vi "CRYPick string arrays to save.vi"(8 "Axes":cluster{"x":bool, "y":bool, "z":bool}, 9 "Layout":enum16{"rows", "columns"}(ring), 10 "Delimiter":string, 11 "Spreadsheet string":string) -> (3 "Spreadsheet string out":string)   [LabVIEW 2013]
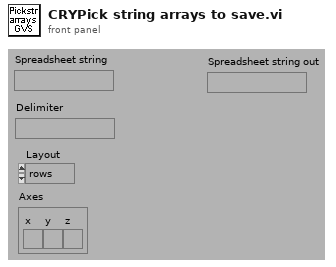
[diagram p1: front panel]
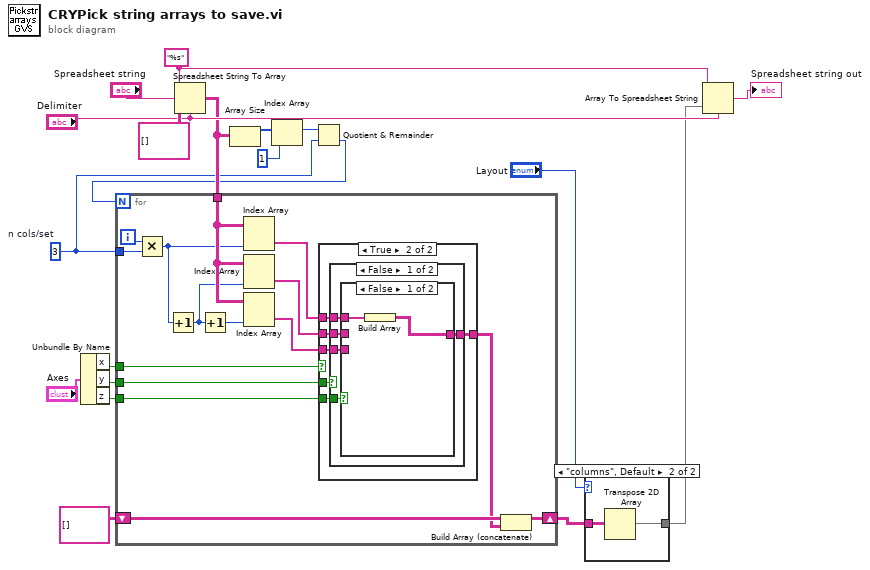
[diagram p0: block diagram]
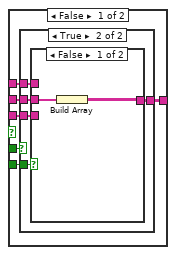
[diagram p3: hidden frame]
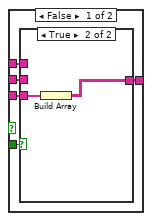
[diagram p4: hidden frame]
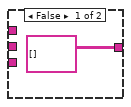
[diagram p5: hidden frame]
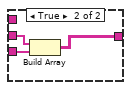
[diagram p6: hidden frame]
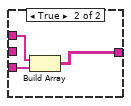
[diagram p7: hidden frame]
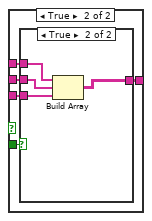
[diagram p8: hidden frame]
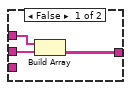
[diagram p9: hidden frame]
diagram:
  w5 = 3  # n cols/set
  w18 = "%s"
  n1 = Unbundle By Name("Axes") -> ("x"=w13:bool, "y"=w12:bool, "z"=w11:bool)
  n2 = Spreadsheet String To Array(delimiter (Tab)="Delimiter", format string=w18, spreadsheet string="Spreadsheet string", array type (2D Dbl)=string[][] []) -> (array=w7:string[][])
  n3 = Array Size(array=w7) -> (size(s)=w9:i32[])
  n4 = Index Array(array=w9, index=1 ("Index")) -> (element=w8:i32)
  n5 = Quotient & Remainder(x=w8, y=w5) -> (floor(x/y)=w6:i32)  [unwired: 1 out]
  n6 = for {
    N: w6 -> [_]
    tunnel: w7 -> [w34]
    tunnel: w13 -> [w30]
    tunnel: w12 -> [w29]
    tunnel: w11 -> [w28]
    tunnel: w5 -> [w25]
    shift-right: [w22] -> w3
    shift-left: string[][] [] -> [w21]
    i -> [w24]
    n7 = Multiply(x=w24, y=w25) -> (x*y=w23:i32)
    n8 = Increment(x=w23) -> (x+1=w26:i32)
    n9 = Increment(x=w26) -> (x+1=w27:i32)
    n10 = Index Array(array=w34, index (col)=w23) -> (element=w33:string[])  [unwired: 1 in]
    n11 = Index Array(array=w34, index (col)=w26) -> (element=w32:string[])  [unwired: 1 in]
    n12 = Index Array(array=w34, index (col)=w27) -> (element=w31:string[])  [unwired: 1 in]
    n13 = case shown="True" w30 {
      tunnel: w29 -> [w40 w64]
      tunnel: w28 -> [w39 w63]
      tunnel: w33 -> [w38 w62]
      tunnel: w32 -> [w37 w61]
      tunnel: w31 -> [w36 w60]
      tunnel: [w35 w59] -> w20
      frame False {
        n14 = case shown="True" w40 {
          tunnel: w39 -> [w45 w53]
          tunnel: w38 -> [w44 w52]
          tunnel: w37 -> [w43 w51]
          tunnel: w36 -> [w42 w50]
          tunnel: [w41 w49] -> w35
          frame False {
            n15 = case shown="True" w45 {
              tunnel: w44 -> [_ _]
              tunnel: w43 -> [_ _]
              tunnel: w42 -> [_ w48]
              tunnel: [string[][] [] w47] -> w41
              frame False {
              }
              frame True {
                n16 = Build Array(w48) -> (w47:string[][])
              }
            }
          }
          frame True {
            n17 = case shown="False" w53 {
              tunnel: w52 -> [_ _]
              tunnel: w51 -> [w55 w56]
              tunnel: w50 -> [_ w58]
              tunnel: [w54 w57] -> w49
              frame False {
                n18 = Build Array(w55) -> (w54:string[][])
              }
              frame True {
                n19 = Build Array(w56, w58) -> (w57:string[][])
              }
            }
          }
        }
      }
      frame True {
        n20 = case shown="False" w64 {
          tunnel: w63 -> [w69 w79]
          tunnel: w62 -> [w68 w78]
          tunnel: w61 -> [w67 w77]
          tunnel: w60 -> [w66 w76]
          tunnel: [w65 w75] -> w59
          frame False {
            n21 = case shown="False" w69 {
              tunnel: w68 -> [w71 w72]
              tunnel: w67 -> [_ _]
              tunnel: w66 -> [_ w74]
              tunnel: [w70 w73] -> w65
              frame False {
                n22 = Build Array(w71) -> (w70:string[][])
              }
              frame True {
                n23 = Build Array(w72, w74) -> (w73:string[][])
              }
            }
          }
          frame True {
            n24 = case shown="True" w79 {
              tunnel: w78 -> [w80 w83]
              tunnel: w77 -> [w82 w84]
              tunnel: w76 -> [_ w86]
              tunnel: [w81 w85] -> w75
              frame False {
                n25 = Build Array(w80, w82) -> (w81:string[][])
              }
              frame True {
                n26 = Build Array(w83, w84, w86) -> (w85:string[][])
              }
            }
          }
        }
      }
    }
    n27 = Build Array (concatenate)(w21, w20) -> (w22:string[][])
  }
  n28 = case shown="\"columns\", Default" "Layout" {
    tunnel: w3 -> [w87 w89]
    tunnel: [w87 w88] -> w2
    frame "rows" {
    }
    frame "columns", Default {
      n29 = Transpose 2D Array(2D array=w89) -> (transposed array=w88:string[][])
    }
  }
  n30 = Array To Spreadsheet String(delimiter (Tab)="Delimiter", array=w2, 3:w18) -> (spreadsheet string=→"Spreadsheet string out":string)
